vi "Clear VI History.vi"   [LabVIEW 2011]
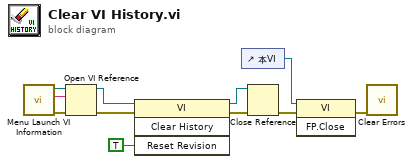
[diagram p0: block diagram]
diagram:
  n1 = call <vilib>:"Menu Launch VI Information.vi"() -> ("error out"=w11:errorcluster, "Menu Launch:VI"=w9:string, "Menu Launch:App"=w10:refnum<vi>)  [unwired: 9 in]
  n2 = Open VI Reference(application reference (local)=w10, vi path=w9, error in (no error)=w11) -> (vi reference=w8:refnum<vi>, error out=w7:errorcluster)  [unwired: 3 in]
  n3 = invoke class="VI" method="Clear History"(reference=w8, error in=w7, "Reset Revision"=TRUE ("重置修订历史")) -> (reference out=w5:refnum<vi>, error out=w4:errorcluster)  [unwired: 1 in, 2 out]
  n4 = control-ref of="本VI"() -> (w2:refnum<vi>)
  n5 = Close Reference(reference=w5, error in (no error)=w4) -> (error out=w3:errorcluster)
  n6 = invoke class="VI" method="FP.Close"(reference=w2, error in=w3) -> (error out=w1:errorcluster)  [unwired: 1 in, 2 out]
  n7 = call <vilib>:"Clear Errors.vi"("error in (no error)"=w1) -> ()  [unwired: 6 in, 1 out]
